vi "LoadClassFromName_Interface.vi"(8 "error in (no error)":errorcluster, 9 "AdditionalData":variant, 10 "Class":string, 11 "iClassLoader In":refnum<class "iClassLoader.lvclass">) -> (0 "error out":errorcluster, 3 "iClassLoader Out":refnum<class "iClassLoader.lvclass">)   [LabVIEW 2020, in "ClassLoader_API.lvlib"]
uses:
  ClassLoader_API.lvlib
  iClassLoader/iClassLoader.lvclass
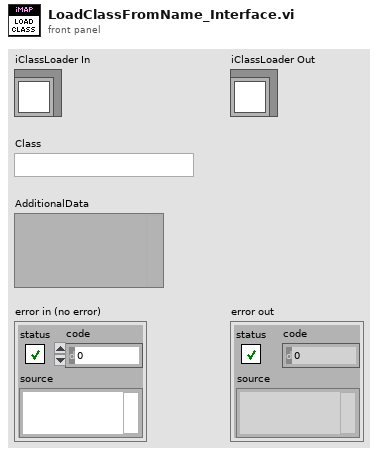
[diagram p1: front panel]
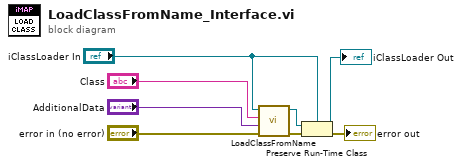
[diagram p0: block diagram]
diagram:
  n1 = call-dynamic "LoadClassFromName.vi"("error in (no error)"="error in (no error)", "AdditionalData"="AdditionalData", "Class"="Class", "iClassLoader in"="iClassLoader In") -> ("error out"=w5:errorcluster, "iClassLoader out"=w3:refnum<class "iClassLoader.lvclass">)  [unwired: 6 in]
  n2 = Preserve Run-Time Class(object in=w3, error in=w5, 2:"iClassLoader In") -> (object out=→"iClassLoader Out":refnum<class "iClassLoader.lvclass">, error out=→"error out":errorcluster)
